vi "Save_Tomography_Data_Main_v2.vi"(8 "error in":errorcluster, 9 "Save CYCLOPS data (?)":bool, 10 "Save raw data (?)":bool, 11 "Data Raw":dbl[][](array[numeric])) -> (0 "error out":errorcluster, 3 "Data CYCLOPS":dbl[][](array[numeric]))   [LabVIEW 2021]
uses:
  <vilib>/Utility/file.llb/Write Delimited Spreadsheet (DBL).vi
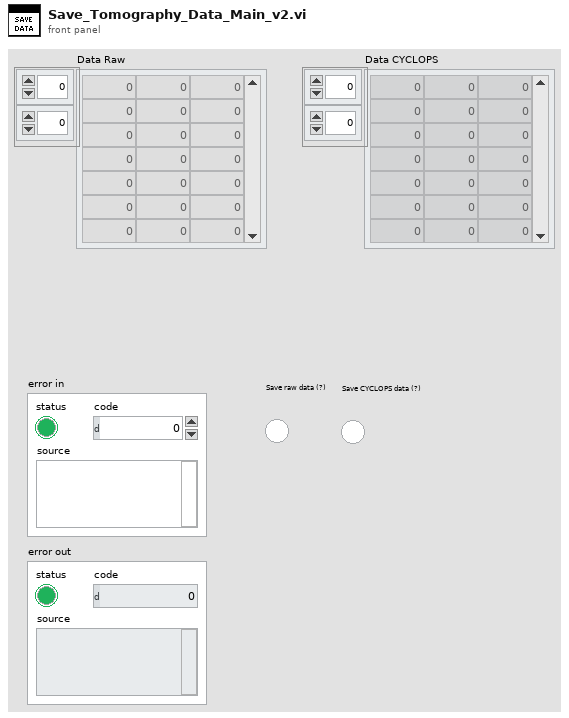
[diagram p1: front panel]
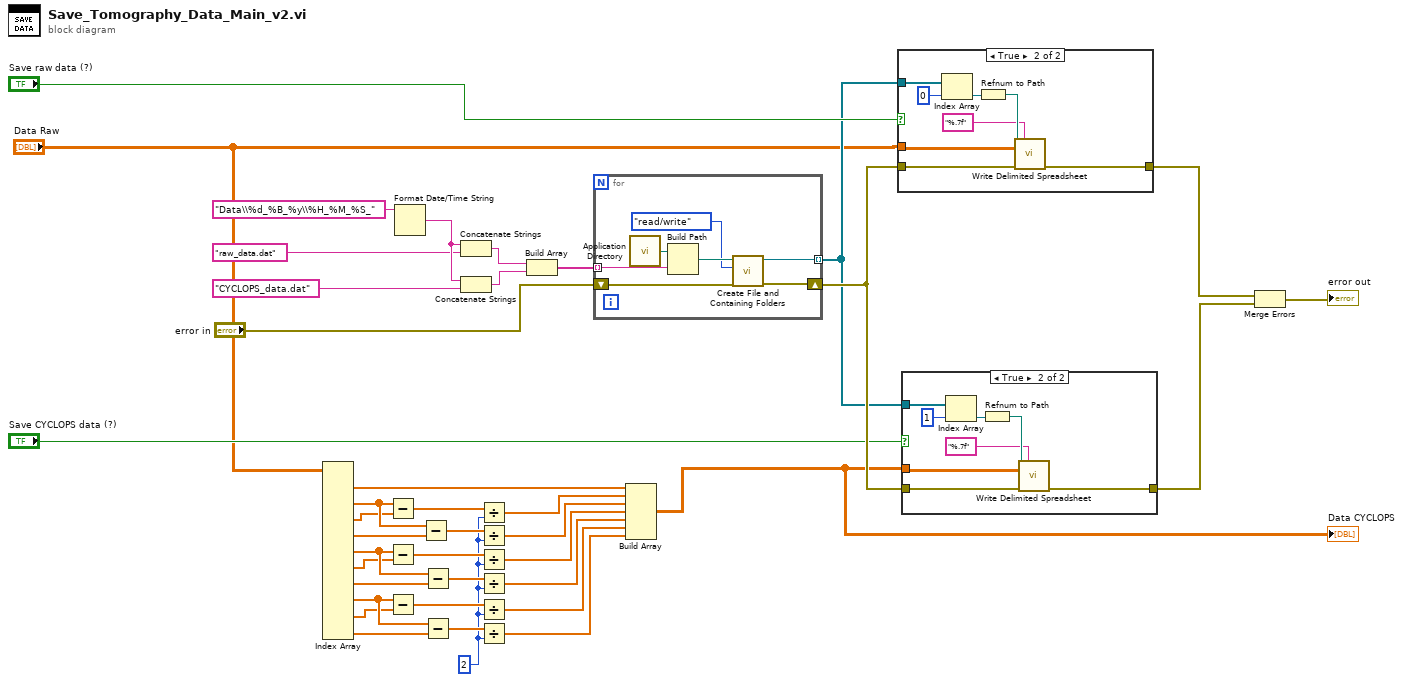
[diagram p0: block diagram]
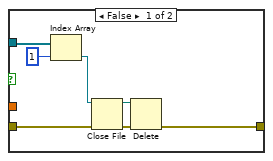
[diagram p2: hidden frame]
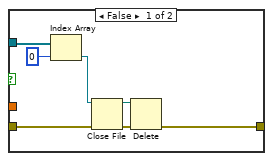
[diagram p3: hidden frame]
diagram:
  w7 = 2
  n1 = Index Array(array="Data Raw") -> (element #1=w22:dbl[], element #2=w21:dbl[], element #3=w20:dbl[], element #4=w23:dbl[], element #5=w19:dbl[], element #6=w18:dbl[], element #7=w17:dbl[], element #8=w16:dbl[], element #9=w14:dbl[], element #10=w15:dbl[])  [unwired: 20 in]
  n2 = Subtract(x=w21, y=w20) -> (x-y=w13:dbl[])
  n3 = Subtract(x=w19, y=w18) -> (x-y=w9:dbl[])
  n4 = Subtract(x=w16, y=w14) -> (x-y=w11:dbl[])
  n5 = Format Date/Time String(time format string (%c)="Data\\%d_%B_%y\\%H_%M_%S_") -> (date/time string=w39:string)  [unwired: 2 in]
  n6 = Subtract(x=w21, y=w23) -> (x-y=w12:dbl[])
  n7 = Subtract(x=w19, y=w17) -> (x-y=w8:dbl[])
  n8 = Subtract(x=w16, y=w15) -> (x-y=w10:dbl[])
  n9 = Concatenate Strings(w39, "raw_data.dat") -> (w36:string)
  n10 = Concatenate Strings(w39, "CYCLOPS_data.dat") -> (w35:string)
  n11 = Divide(x=w13, y=w7) -> (x/y=w1:dbl[])
  n12 = Divide(x=w12, y=w7) -> (x/y=w2:dbl[])
  n13 = Divide(x=w9, y=w7) -> (x/y=w3:dbl[])
  n14 = Divide(x=w8, y=w7) -> (x/y=w4:dbl[])
  n15 = Divide(x=w11, y=w7) -> (x/y=w5:dbl[])
  n16 = Divide(x=w10, y=w7) -> (x/y=w6:dbl[])
  n17 = Build Array(w36, w35) -> (w34:string[])
  n18 = for {
    tunnel: [w41] -> w30 mode=indexing
    tunnel: w34 -> [w44] mode=indexing
    shift-right: [w42] -> w31
    shift-left: "error in" -> [w43]
    n19 = call <vilib>:"Application Directory.vi"() -> ("Application Directory"=w46:path)
    n20 = Build Path(base path=w46, name or relative path=w44) -> (appended path=w47:path)
    n21 = call <vilib>:"Create File and Containing Folders.vi"("error in (no error)"=w43, "access"=enum16{"read/write", "read-only", "write-only"}."read/write", "file path"=w47) -> ("error out"=w42:errorcluster, "refnum out"=w41:refnum<file>)  [unwired: 7 in]
  }
  n22 = Build Array(w22, w1, w2, w3, w4, w5, w6) -> (w24:dbl[][])
  "Data CYCLOPS" <- w24
  n23 = case shown="True" "Save raw data (?)" {
    tunnel: w30 -> [w53 w61]
    tunnel: "Data Raw" -> [_ w60]
    tunnel: w31 -> [w49 w59]
    tunnel: [w52 w58] -> w29
    frame False {
      n24 = Index Array(array=w53, index=0) -> (element=w50:refnum<file>)
      n25 = Close File(refnum=w50, error in=w49) -> (path=w51:path, error out=w48:errorcluster)
      n26 = Delete(path (use dialog)=w51, error in=w48) -> (error out=w52:errorcluster)  [unwired: 3 in, 2 out]
    }
    frame True {
      n27 = Index Array(array=w61, index=0) -> (element=w57:refnum<file>)
      n28 = Refnum to Path(1:w57) -> (0:w56:path)
      n29 = call-poly <vilib>:"Write Delimited Spreadsheet.vi"("file path (dialog if empty)"=w56, "format (%.3f)"="%.7f", "2D data"=w60, "error in (no error)"=w59) -> ("error out"=w58:errorcluster)  [unwired: 10 in, 1 out]
    }
  }
  n30 = case shown="True" "Save CYCLOPS data (?)" {
    tunnel: w30 -> [w68 w76]
    tunnel: w24 -> [_ w75]
    tunnel: w31 -> [w64 w74]
    tunnel: [w67 w73] -> w28
    frame False {
      n31 = Index Array(array=w68, index=1) -> (element=w65:refnum<file>)
      n32 = Close File(refnum=w65, error in=w64) -> (path=w66:path, error out=w63:errorcluster)
      n33 = Delete(path (use dialog)=w66, error in=w63) -> (error out=w67:errorcluster)  [unwired: 3 in, 2 out]
    }
    frame True {
      n34 = Index Array(array=w76, index=1) -> (element=w72:refnum<file>)
      n35 = Refnum to Path(1:w72) -> (0:w71:path)
      n36 = call-poly <vilib>:"Write Delimited Spreadsheet.vi"("file path (dialog if empty)"=w71, "format (%.3f)"="%.7f", "2D data"=w75, "error in (no error)"=w74) -> ("error out"=w73:errorcluster)  [unwired: 10 in, 1 out]
    }
  }
  n37 = Merge Errors(w29, w28) -> (→"error out":errorcluster)
